vi "testControlNotOnConnectorPane.vi"() -> ()   [LabVIEW 2017, in "Theory.Tests.lvlib"]
uses:
  Theory.Tests.lvlib
  ControlData.ctl
  Theory/Theory.lvclass
  Assertion/Assertion.lvlib
  Support/Support.lvlib
panel:
  out "error out":errorcluster
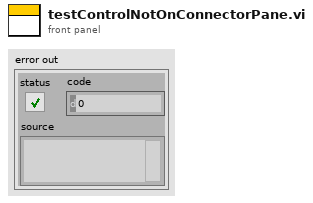
[diagram p1: front panel]
types:
  T1 = typedef "ControlData.ctl" = cluster{"Name":string, "Data":variant}
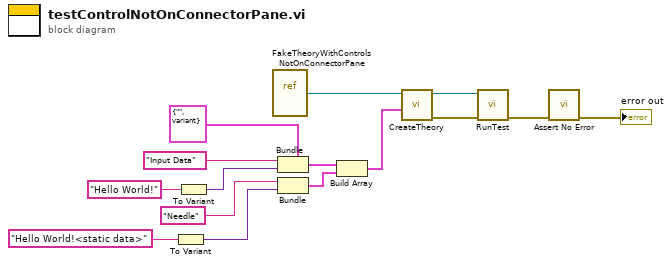
[diagram p0: block diagram]
diagram:
  n1 = To Variant(anything="Hello World!<static data>" ("key")) -> (Variant=w3:variant)
  n2 = To Variant(anything="Hello World!" ("key")) -> (Variant=w9:variant)
  n3 = vi-ref "FakeTheoryWithControlsNotOnConnectorPane.vi"() -> (w6:refnum<vi>)
  n4 = Bundle(cluster=T1 {"Name"="", "Data"=variant} ("Control Data"), "Name"="Input Data" ("key"), "Data"=w9) -> (w10:T1)
  n5 = Bundle("key"="Needle", "Variant"=w3) -> (w1:cluster{"key":string, "Variant":variant})  [unwired: 1 in]
  n6 = Build Array(w10, w1) -> (w2:T1[])
  n7 = call "CreateTheory.vi"("Control Data"=w2, "VI Refnum"=w6) -> ("error out"=w14:errorcluster, "Theory"=w15:refnum<class "Theory.lvclass">)  [unwired: 8 in]
  n8 = call-dynamic "RunTest.vi"("error in (no error)"=w14, "Theory in"=w15) -> ("error out"=w13:errorcluster)  [unwired: 8 in, 1 out]
  n9 = call "Assert No Error.vi"("error in (no error)"=w13) -> ("error out"=→"error out":errorcluster)  [unwired: 10 in]
